vi "lvcsm List Sesctions.vi"(6 "Config Path":path, 8 "error in (no error)":errorcluster) -> (0 "error out":errorcluster, 3 "Section Names":string[](array[string]))   [LabVIEW 2017, in "lvcsm File Support.lvlib"]
uses:
  lvcsm File Support.lvlib
  <vilib>/Utility/config.llb/NI_LVConfig.lvlib
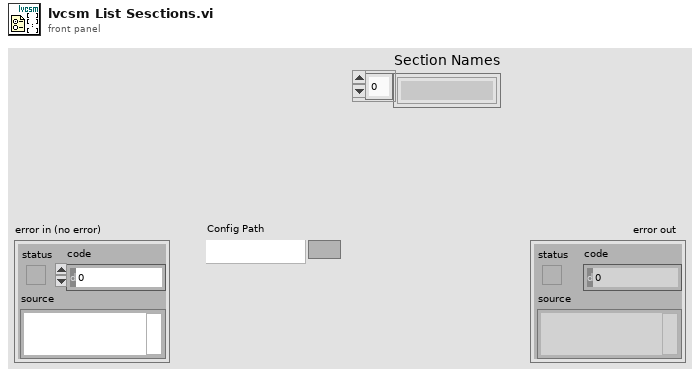
[diagram p1: front panel]
types:
  T1 = typedef "NI_LVConfig.lvlib/Config Data RefNum.ctl" = refnum<k1>
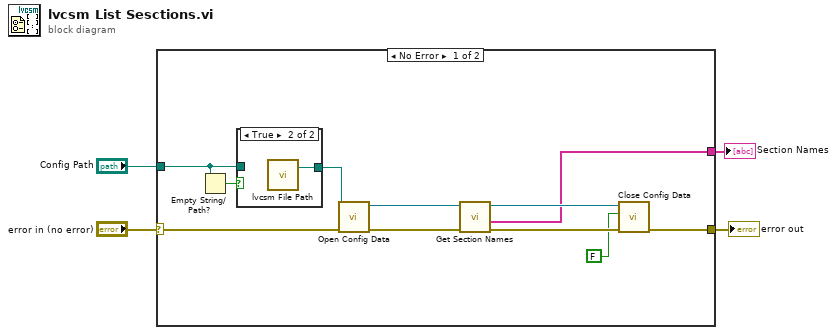
[diagram p0: block diagram]
diagram:
  n1 = case shown="No Error" "error in (no error)" {
    selector: "error in (no error)" -> [w13 w18]
    tunnel: "Config Path" -> [w15 _]
    tunnel: [w14 w18] -> w2
    tunnel: [w5 _] -> w1
    frame No Error {
      n2 = Empty String/Path?(string/path=w15) -> (empty?=w12:bool)
      n3 = case shown="True" w12 {
        tunnel: [w16 w17] -> w11
        tunnel: w15 -> [w16 _]
        frame False {
        }
        frame True {
          n4 = call "lvcsm File Path.vi"() -> ("Appended Path"=w17:path)  [unwired: 3 in]
        }
      }
      n5 = call <vilib>:"Open Config Data.vi"("error in (no error)"=w13, "configuration file path"=w11) -> ("error out"=w9:errorcluster, "refnum"=w10:T1)  [unwired: 7 in, 1 out]
      n6 = call <vilib>:"Get Section Names.vi"("error in (no error)"=w9, "refnum"=w10) -> ("error out"=w8:errorcluster, "section names"=w5:string[], "refnum out"=w7:T1)  [unwired: 7 in]
      n7 = call <vilib>:"Close Config Data.vi"("error in (no error)"=w8, "write file if changed (T)"=FALSE, "refnum"=w7) -> ("error out"=w14:errorcluster)  [unwired: 7 in, 1 out]
    }
    frame Error {
    }
  }
  "error out" <- w2
  "Section Names" <- w1
